vi "client.vi"   [LabVIEW 2014]
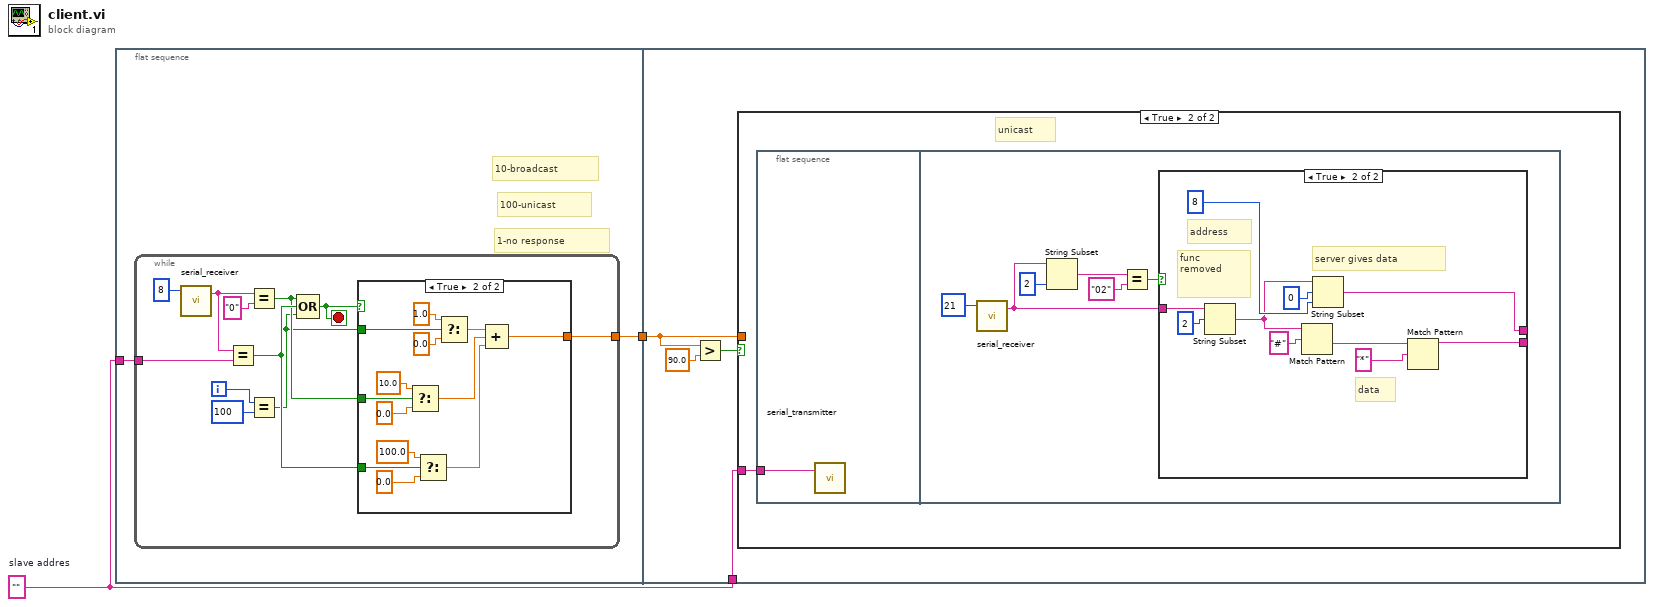
[diagram p0: block diagram]
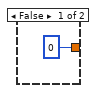
[diagram p2: hidden frame]
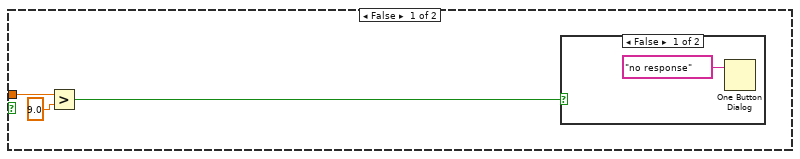
[diagram p3: hidden frame]
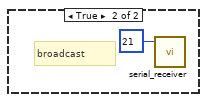
[diagram p4: hidden frame]
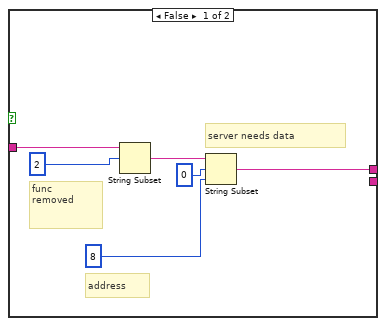
[diagram p5: hidden frame]
diagram:
  w1 = ""  # slave addres
  n1 = flat-sequence {
    tunnel: w1 -> [w4]
    tunnel: [w3] -> w2
    tunnel: w2 -> [w30]
    tunnel: w1 -> [w31]
    frame #0 {
      # "10-broadcast"
      # "100-unicast"
      # "1-no response"
      n2 = while {
        tunnel: w4 -> [w12]
        tunnel: [w5] -> w3
        i -> [w11]
        stop <- w9 stop-if-true
        n3 = call "serial_receiver.vi"("byte count"=u32 8) -> ("read buffer"=w13:string)  [unwired: 1 in, 2 out]
        n4 = Equal?(x=w13, y=w12) -> (x = y?=w8:bool)
        n5 = Equal?(x=w13, y="0") -> (x = y?=w7:bool)
        n6 = Equal?(x=w11, y=100) -> (x = y?=w6:bool)
        n7 = Compound Arithmetic op=OR(w7, w8, w6) -> (w9:bool)
        n8 = case shown="True" w9 {
          tunnel: w8 -> [_ w20]
          tunnel: w7 -> [_ w19]
          tunnel: w6 -> [_ w18]
          tunnel: [0 w17] -> w5
          frame False {
          }
          frame True {
            n9 = Select(t=10.0, s=w19, f=0.0) -> (s? t:f=w28:dbl)
            n10 = Select(t=100.0, s=w20, f=0.0) -> (s? t:f=w29:dbl)
            n11 = Select(t=1.0, s=w18, f=0.0) -> (s? t:f=w27:dbl)
            n12 = Compound Arithmetic op=ADD(w27, w28, w29) -> (w17:dbl)
          }
        }
      }
    }
    frame #1 {
      n13 = Greater?(x=w30, y=90.0) -> (0:w32:bool)
      n14 = case shown="True" w32 {
        tunnel: w31 -> [_ w39]
        tunnel: w30 -> [w36 _]
        frame False {
          n15 = Greater?(x=w36, y=9.0) -> (0:w34:bool)
          n16 = case shown="False" w34 {
            frame False {
              n17 = One Button Dialog(message="no response") -> ()  [unwired: 1 in, 1 out]
            }
            frame True {
              # "broadcast"
              n18 = call "serial_receiver.vi"("byte count"=u32 21) -> ()  [unwired: 1 in, 3 out]
            }
          }
        }
        frame True {
          # "unicast"
          n19 = flat-sequence {
            tunnel: w39 -> [w40]
            frame #0 {
              n20 = call "serial_transmitter.vi"("write buffer"=w40) -> ()  [unwired: 1 in, 2 out]
            }
            frame #1 {
              n21 = call "serial_receiver.vi"("byte count"=u32 21) -> ("read buffer"=w41:string)  [unwired: 1 in, 2 out]
              n22 = String Subset(string=w41, length (rest)=2 ("length (rest)")) -> (substring=w44:string)  [unwired: 1 in]
              n23 = Equal?(x=w44, y="02") -> (x = y?=w42:bool)
              n24 = case shown="True" w42 {
                tunnel: w41 -> [w48 w62]
                tunnel: [w47 w58] -> _
                tunnel: [_ w53] -> _
                frame False {
                  # "address"
                  # "func\nremoved"
                  # "server needs data"
                  n25 = String Subset(string=w48, offset (0)=2) -> (substring=w49:string)  [unwired: 1 in]
                  n26 = String Subset(string=w49, offset (0)=0, length (rest)=8 ("length (rest)")) -> (substring=w47:string)
                }
                frame True {
                  # "data"
                  # "address"
                  # "func\nremoved"
                  # "server gives data"
                  n27 = String Subset(string=w62, offset (0)=2) -> (substring=w57:string)  [unwired: 1 in]
                  n28 = Match Pattern(string=w57, regular expression="#") -> (after substring=w54:string)  [unwired: 1 in, 3 out]
                  n29 = String Subset(string=w57, offset (0)=0, length (rest)=8 ("length (rest)")) -> (substring=w58:string)
                  n30 = Match Pattern(string=w54, regular expression="*") -> (before substring=w53:string)  [unwired: 1 in, 3 out]
                }
              }
            }
          }
        }
      }
    }
  }
